vi "_TangoReadBooleanScalarAttribute.vi"(3 "error in":errorcluster, 4 "attribute name":string, 5 "device name":string) -> (0 "error out":errorcluster, 1 "setpoint":bool, 2 "value":bool)   [LabVIEW 2014, in "tango.lvlib"]
uses:
  tango.lvlib
  Common VIs/Typedefs/_AttributeDataType_t.ctl
  Extractors/base/toBooleanScalar.vi
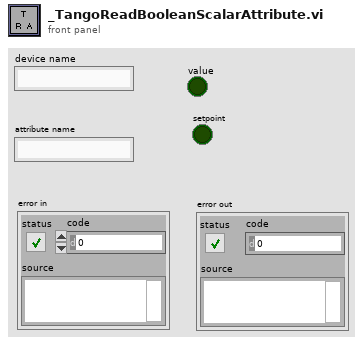
[diagram p1: front panel]
types:
  T1 = typedef "tango.lvlib/_AttributeDataType_t.ctl" = enum16{"STATE_SCA", "STATE_SPE", "STATE_IMG", "STRING_SCA", "STRING_SPE", "STRING_IMG", "BOOL_SCA", "BOOL_SPE", "BOOL_IMG", "UCHAR_SCA", "UCHAR_SPE", "UCHAR_IMG", "SHORT_SCA", "SHORT_SPE", "SHORT_IMG", "USHORT_SCA", "USHORT_SPE", "USHORT_IMG", "LONG_SCA", "LONG_SPE", "LONG_IMG", "ULONG_SCA", "ULONG_SPE", "ULONG_IMG", "LONG64_SCA", "LONG64_SPE", "LONG64_IMG", "ULONG64_SCA", "ULONG64_SPE", "ULONG64_IMG", "FLOAT_SCA", "FLOAT_SPE", "FLOAT_IMG", "DOUBLE_SCA", "DOUBLE_SPE", "DOUBLE_IMG", "UNKNOWN_DATA_TYPE"}
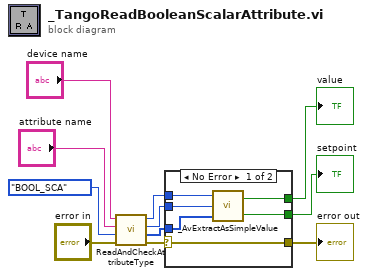
[diagram p0: block diagram]
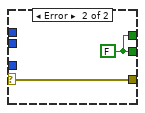
[diagram p2: hidden frame]
diagram:
  n1 = call "ReadAndCheckAttributeType.vi"("error in (no error)"="error in", "expected data type"=_AttributeDataType_t."BOOL_SCA" ("Control"), "attribute name"="attribute name", "device name"="device name") -> ("error out"=w1:errorcluster, "value"=w2:u8[], "dim. y"=w3:i32, "dim. x"=w4:i32)  [unwired: 4 in]
  n2 = case shown="No Error" w1 {
    selector: w1 -> [w12 w18]
    tunnel: w4 -> [w17 _]
    tunnel: w3 -> [w16 _]
    tunnel: w2 -> [w15 _]
    tunnel: [w14 w19] -> w11
    tunnel: [w13 w19] -> w10
    tunnel: [w12 w18] -> w9
    frame No Error {
      n3 = call-poly "_AvExtractAsSimpleValue.vi"("value_in"=w15, "dim_y"=w16, "dim_x"=w17) -> ("setpoint"=w13:bool, "value_out"=w14:bool)
    }
    frame Error {
      w19 = FALSE ("value_out")
    }
  }
  "error out" <- w9
  "value" <- w11
  "setpoint" <- w10
